vi "DAQ Assistant.vi"() -> ()   [LabVIEW 2017]
panel:
  in  "stop":bool
  in  "rate":dbl=1000.0
  in  "number of samples":i32=1000
  out "Waveform Graph":dynamicdata(graph)
  out "error out":errorcluster
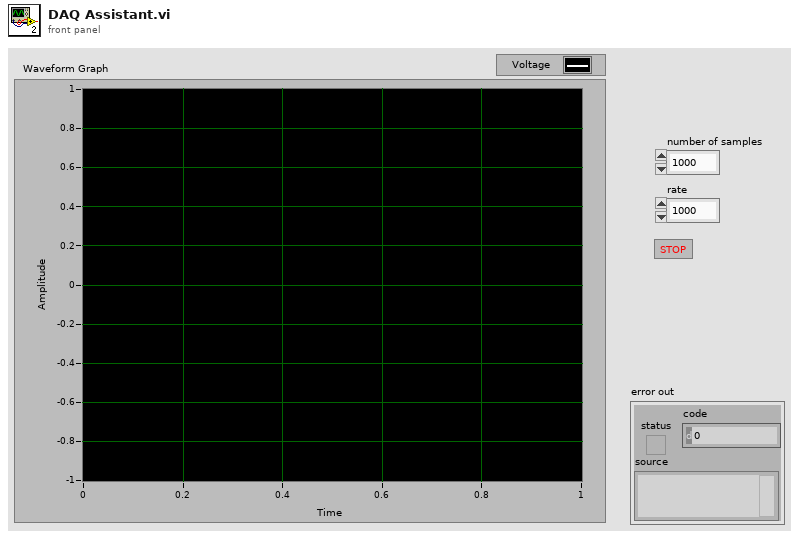
[diagram p1: front panel]
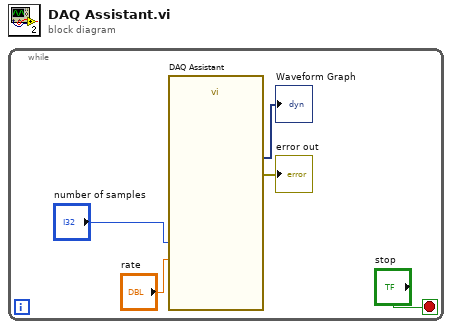
[diagram p0: block diagram]
diagram:
  n1 = while {
    stop <- "stop" stop-if-true
    n2 = call "DAQ Assistant"("rate"="rate", "number of samples"="number of samples") -> ("data"=→"Waveform Graph":dynamicdata, "error out"=→"error out":errorcluster)  [unwired: 15 in, 1 out]
  }
